vi "Recall Data From File.vi"(4 "Waveform Generator (0: Waveform Generator 1)":i32(ring) items=["Waveform Generator 1", "Waveform Generator 2"], 6 "Arbitrary Column Number (1)":i32=1, 7 "Internal Location":string, 8 "error in (no error)":errorcluster, 9 "Waveform Memory Location (1: Waveform Memory 1)":i32(ring)=1 items=["Waveform Memory 1"=1, "Waveform Memory 2"=2], 10 "File Type (0: Mask)":i32(ring) items=["Mask", "Setup", "Waveform", "Arbitrary"], 11 "VISA resource name":refnum<visa-resource-name>) -> (0 "error out":errorcluster, 3 "VISA resource name out":refnum<visa-resource-name>)   [LabVIEW 2010, in "Agilent 2000 3000 X-Series.lvlib"]
doc: "Configure the recall file operation."
uses:
  <instrlib>/Agilent 2000 3000 X-Series/Agilent 2000 3000 X-Series.lvlib
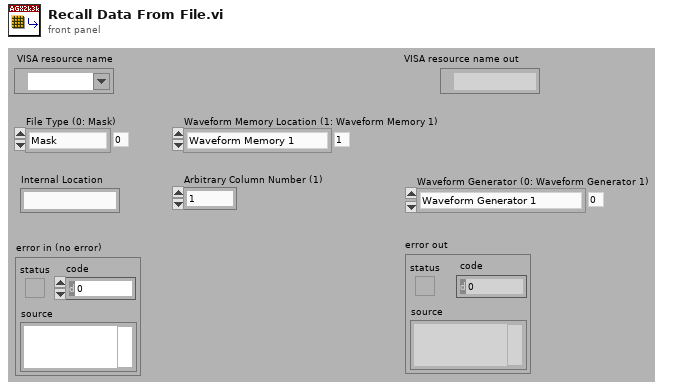
[diagram p1: front panel]
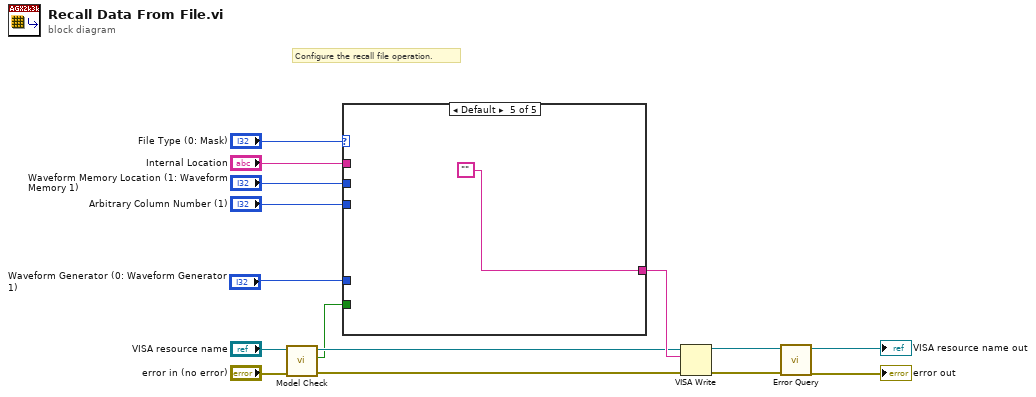
[diagram p0: block diagram]
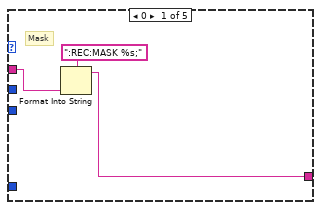
[diagram p2: hidden frame]
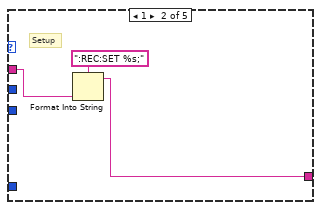
[diagram p3: hidden frame]
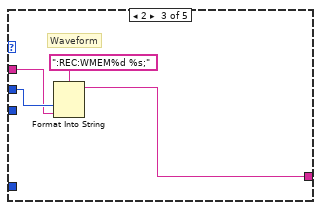
[diagram p4: hidden frame]
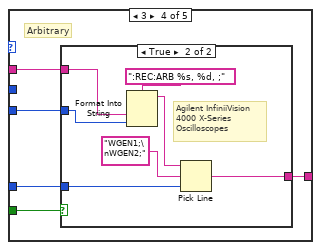
[diagram p5: hidden frame]
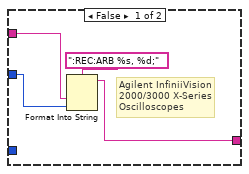
[diagram p6: hidden frame]
diagram:
  # "Configure the recall file operation."
  n1 = call <instrlib>:"Model Check.vi"("error in (no error)"="error in (no error)", "VISA resource name"="VISA resource name") -> ("error out"=w2:errorcluster, "Is 4000 Series"=w1:bool, "VISA resource name out"=w3:refnum<visa-resource-name>)  [unwired: 7 out]
  n2 = case shown="Default" "File Type (0: Mask)" {
    tunnel: "Internal Location" -> [w18 w20 w23 w30 _]
    tunnel: "Waveform Memory Location (1: Waveform Memory 1)" -> [_ _ w24 _ _]
    tunnel: [w16 w19 w22 w28 ""] -> w8
    tunnel: "Arbitrary Column Number (1)" -> [_ _ _ w29 _]
    tunnel: "Waveform Generator (0: Waveform Generator 1)" -> [_ _ _ w27 _]
    tunnel: w1 -> [_ _ _ w26 _]
    frame 0 {
      # "Mask"
      n3 = Format Into String(format string=":REC:MASK %s;", w18) -> (resulting string=w16:string)  [unwired: 2 in, 1 out]
    }
    frame 1 {
      # "Setup"
      n4 = Format Into String(format string=":REC:SET %s;", w20) -> (resulting string=w19:string)  [unwired: 2 in, 1 out]
    }
    frame 2 {
      # "Waveform"
      n5 = Format Into String(format string=":REC:WMEM%d %s;", w24, w23) -> (resulting string=w22:string)  [unwired: 2 in, 1 out]
    }
    frame 3 {
      # "Arbitrary"
      n6 = case shown="True" w26 {
        tunnel: w30 -> [w34 w40]
        tunnel: w29 -> [w33 w39]
        tunnel: [w32 w35] -> w28
        tunnel: w27 -> [_ w36]
        frame False {
          # "Agilent InfiniiVision\n2000/3000 X-Series\nOscilloscopes"
          n7 = Format Into String(format string=":REC:ARB %s, %d;", w34, w33) -> (resulting string=w32:string)  [unwired: 2 in, 1 out]
        }
        frame True {
          # "Agilent InfiniiVision\n4000 X-Series\nOscilloscopes"
          n8 = Format Into String(format string=":REC:ARB %s, %d, ;", w40, w39) -> (resulting string=w38:string)  [unwired: 2 in, 1 out]
          n9 = Pick Line(string ("")=w38, multi-line string="WGEN1;\nWGEN2;", line index=w36) -> (output string=w35:string)
        }
      }
    }
    frame Default {
    }
  }
  n10 = VISA Write(VISA resource name=w3, write buffer=w8, error in (no error)=w2) -> (VISA resource name out=w15:refnum<visa-resource-name>, error out=w14:errorcluster)  [unwired: 1 out]
  n11 = call <instrlib>:"Error Query.vi"("error in (no error)"=w14, "VISA resource name"=w15) -> ("error out"=→"error out":errorcluster, "VISA resource name out"=→"VISA resource name out":refnum<visa-resource-name>)  [unwired: 8 out]
